vi "TachoTest.vi"() -> ()   [LabVIEW 2023]
uses:
  <vilib>/DAQmx/read.llb/DAQmx Read (Digital Wfm 1Chan NSamp).vi
  <vilib>/DAQmx/create/channels.llb/DAQmx Create Channel (DI-Digital Input).vi
  <vilib>/DAQmx/configure/timing.llb/DAQmx Timing (Sample Clock).vi
  <vilib>/DAQmx/miscellaneous.llb/DAQmx Fill In Error Info.vi
  <vilib>/Waveform/DTblOps.llb/DTbl Digital to Binary U32.vi
  <resource>/objmgr/daqmx.rc
  <vilib>/addons/Sound and Vibration/Order Analysis/Tach Process/SoundVib_TachProcess.lvlib
panel:
  in  "# samples per capture":i32=1000
  out "Digital Waveform Graph":digitalwaveform(graph)
  in  "Mode":enum16{"Continuous", "Finite (manual trigger)"}(ring)
  in  "Sample rate (Hz)":dbl=1000.0
  out "Actual Sample Rate":dbl=1000.0 format="%0.2f"
  in  "Line(s)":tag="Dev1/port0/line0:7"
  out "size(s)":i32
  out "Current time stamp":timestamp format="%<%x %.3X>T"
  out "Data":digitaldata
  out "dt":dbl
  out "Capture complete":bool
  out "t0":timestamp
  in  "StopVI":bool
  in  "CaptureButton":bool
  # "IO Setup"
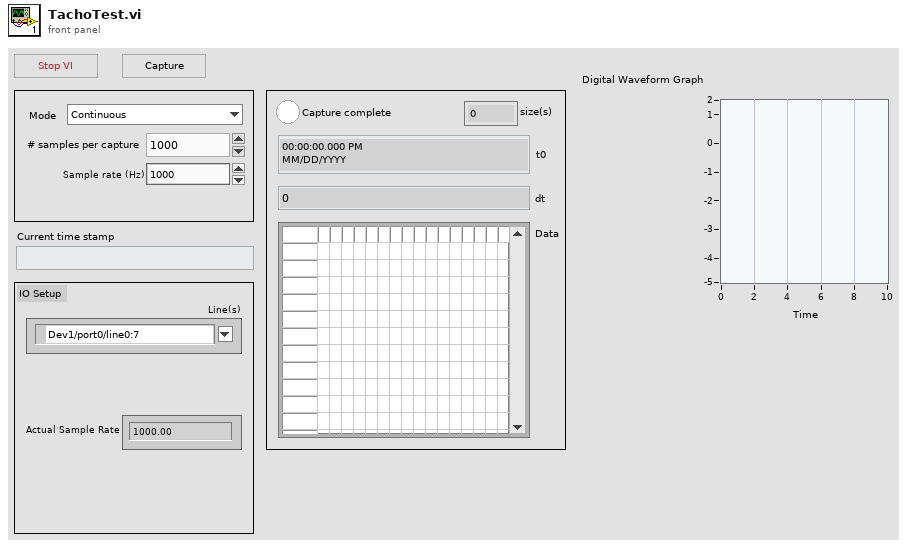
[diagram p1: front panel]
types:
  T1 = enum8{"Enabled", "Disabled", "Disabled and Grayed Out"}
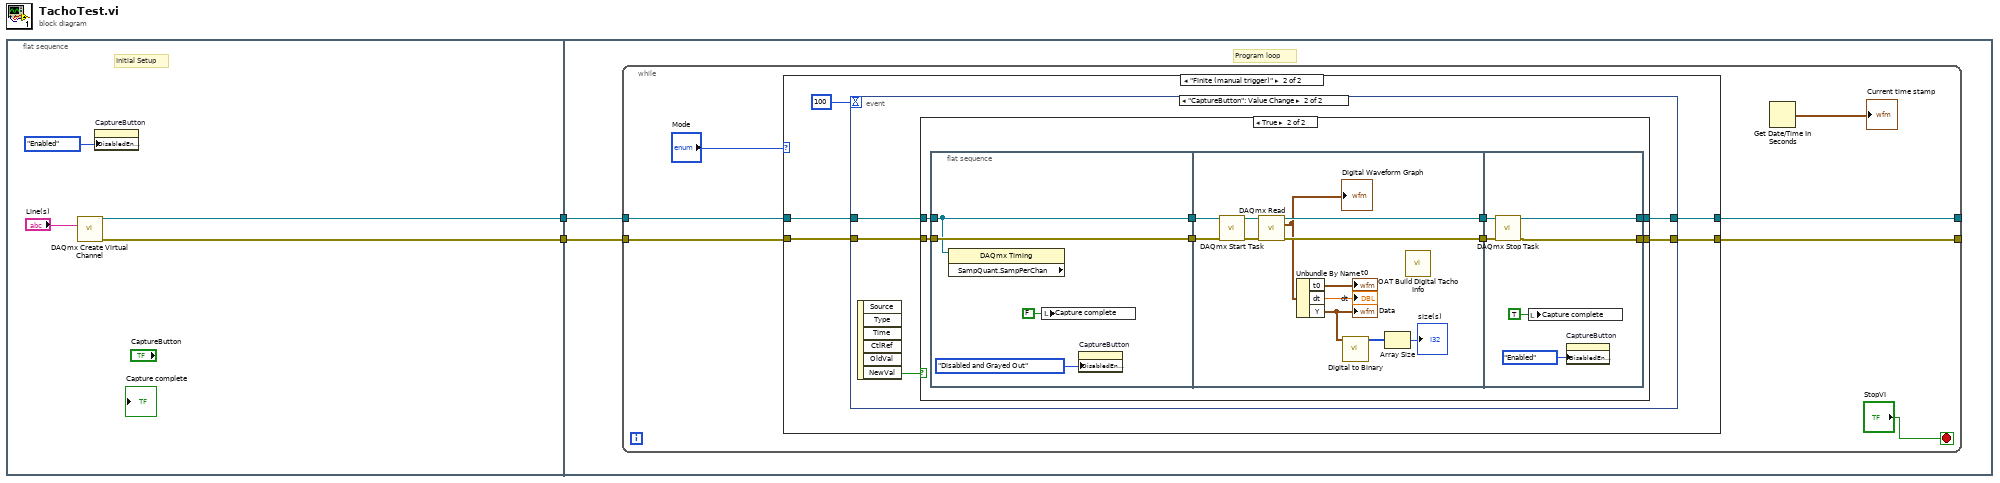
[diagram p0: block diagram]
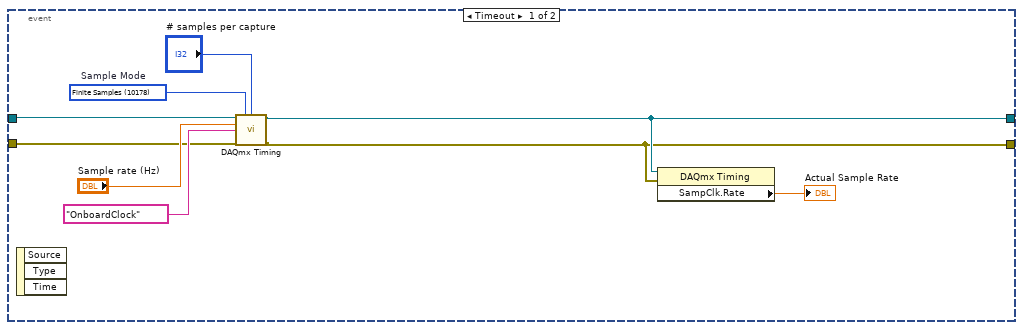
[diagram p3: hidden frame]
diagram:
  n1 = flat-sequence {
    tunnel: [w3] -> w2
    tunnel: [w4] -> w1
    tunnel: w2 -> [w7]
    tunnel: w1 -> [w8]
    frame #0 {
      # "Initial Setup"
      n2 = call-poly <vilib>:"DAQmx Create Virtual Channel.vi"("lines"="Line(s)") -> ("task out"=w4:refnum<k21>, "error out"=w3:errorcluster)  [unwired: 13 in]
      n3 = property on="CaptureButton" class="Bool (strict)"("DisabledEnum"=T1."Enabled" ("Disabled")) -> ()  [unwired: 2 in, 2 out]
    }
    frame #1 {
      # "Program loop"
      n4 = while {
        tunnel: w8 -> [w13]
        tunnel: w7 -> [w12]
        tunnel: [w11] -> _
        tunnel: [w10] -> _
        stop <- "StopVI" stop-if-true
        n5 = case shown="\"Finite (manual trigger)\"" "Mode" {
          tunnel: w13 -> [w17 w22]
          tunnel: w12 -> [w16 w21]
          tunnel: [w17 w20] -> w11
          tunnel: [w16 w19] -> w10
          frame "Continuous", Default {
          }
          frame "Finite (manual trigger)" {
            n6 = event shown="[1] \"CaptureButton\": Value Change" {
              selector: _ -> [_ _]
              dyn-events: _ -> [_ _]
              timeout: 100 -> [_ _]
              tunnel: w22 -> [w26 w35]
              tunnel: w21 -> [w24 w34]
              tunnel: [w25 w33] -> w20
              tunnel: [w23 w32] -> w19
              event Timeout {
                w28 = 10178 items=["Finite Samples"=10178, "Continuous Samples"=10123, "Hardware Timed Single Point"=12522]  # Sample Mode
                n7 = event-data() -> ()  [unwired: 1 in, 3 out]
                n8 = call-poly <vilib>:"DAQmx Timing.vi"("task/channels in"=w26, "sample mode"=w28, "samples per channel"="# samples per capture", "rate"="Sample rate (Hz)", "source"=tag "OnboardClock", "error in"=w24) -> ("task out"=w25:refnum<k21>, "error out"=w23:errorcluster)  [unwired: 8 in]
                n9 = property class="DAQmx Timing"(reference=w25, error in=w23) -> ("SampClk.Rate"=→"Actual Sample Rate":dbl)  [unwired: 2 out]
              }
              event "CaptureButton": Value Change {
                n10 = event-data() -> ("NewVal"=w36:bool)  [unwired: 1 in, 5 out]
                n11 = case shown="True" w36 {
                  tunnel: w35 -> [w38 w46]
                  tunnel: w34 -> [w37 w45]
                  tunnel: [w38 w40] -> w33
                  tunnel: [w37 w39] -> w32
                  frame False {
                  }
                  frame True {
                    n12 = flat-sequence {
                      tunnel: w45 -> [w50]
                      tunnel: w46 -> [w47]
                      tunnel: [w47] -> w42
                      tunnel: [w50] -> w41
                      tunnel: [w53] -> w44
                      tunnel: [w52] -> w43
                      tunnel: w42 -> [w62]
                      tunnel: w41 -> [w61]
                      tunnel: w44 -> [w68]
                      tunnel: w43 -> [w67]
                      tunnel: [w64] -> w40
                      tunnel: [w63] -> w39
                      frame #0 {
                        n13 = property class="DAQmx Timing" props=["SampQuant.SampPerChan"](reference=w47) -> ()  [unwired: 1 in, 3 out]
                        n14 = local write "Capture complete"(FALSE ("Capture complete")) -> ()
                        n15 = property on="CaptureButton" class="Bool (strict)"("DisabledEnum"=T1."Disabled and Grayed Out" ("Disabled")) -> ()  [unwired: 2 in, 2 out]
                      }
                      frame #1 {
                        n16 = call <vilib>:"DAQmx Start Task.vi"("task/channels in"=w62, "error in"=w61) -> ("task out"=w60:refnum<k21>, "error out"=w59:errorcluster)  [unwired: 12 in]
                        n17 = call-poly <vilib>:"DAQmx Read.vi"("task/channels in"=w60, "error in"=w59) -> ("task out"=w53:refnum<k21>, "data"=w51:digitalwaveform, "error out"=w52:errorcluster)  [unwired: 11 in]
                        "Digital Waveform Graph" <- w51
                        n18 = Unbundle By Name(w51) -> ("t0"=→"t0":timestamp, "dt"=→"dt":dbl, "Y"=w55:digitaldata)
                        "Data" <- w55
                        n19 = call-poly <vilib>:"Digital to Binary.vi"("digital data"=w55) -> ("binary array"=w54:u32[])  [unwired: 9 in, 1 out]
                        n20 = Array Size(array=w54) -> (size(s)=→"size(s)":i32)
                        n21 = call <vilib>:"OAT Build Digital Tacho Info.vi"() -> ()  [unwired: 14 in, 2 out]
                      }
                      frame #2 {
                        n22 = call <vilib>:"DAQmx Stop Task.vi"("task/channels in"=w68, "error in"=w67) -> ("task out"=w64:refnum<k21>, "error out"=w63:errorcluster)  [unwired: 12 in]
                        n23 = local write "Capture complete"(TRUE ("Capture complete")) -> ()
                        n24 = property on="CaptureButton" class="Bool (strict)"("DisabledEnum"=T1."Enabled" ("Disabled")) -> ()  [unwired: 2 in, 2 out]
                      }
                    }
                  }
                }
              }
            }
          }
        }
        n25 = Get Date/Time In Seconds() -> (seconds since 1Jan1904=→"Current time stamp":timestamp)
      }
    }
  }
